vi "Get Default Pressure Units.vi"(8 "error in (no error)":errorcluster, 11 "VISA resource name":refnum<visa-resource-name>) -> (0 "error out":errorcluster, 2 "Default Pressure Units":i32, 3 "VISA resource name out":refnum<visa-resource-name>)   [LabVIEW 2013, in "Fluke 5XXX Series Multicalibrators.lvlib"]
doc: "This VI returns the power-up and reset default pressure display units.\n\nNote:\n\nThis VI is available only for instrument model 5520A with option 700P (pressure modules)."
uses:
  Fluke 5XXX Series Multicalibrators.lvlib
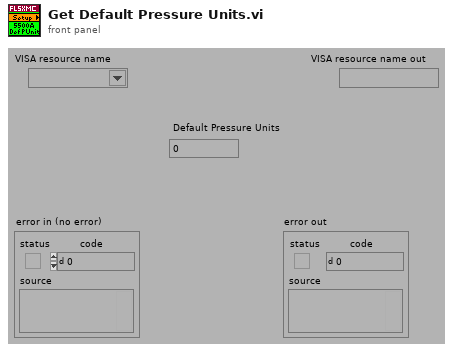
[diagram p1: front panel]
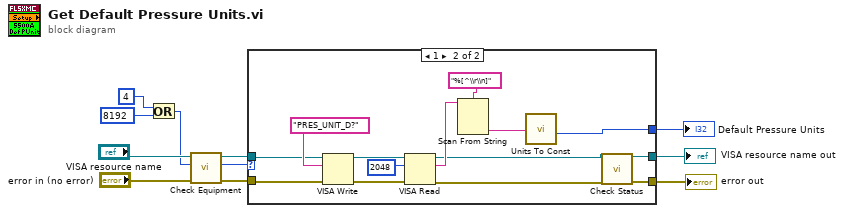
[diagram p0: block diagram]
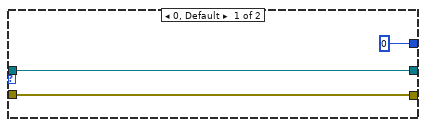
[diagram p2: hidden frame]
diagram:
  n1 = Or(x=4 ("Numeric"), y=8192 ("Numeric")) -> (x .or. y?=w2:i32)
  n2 = call "Check Equipment.vi"("error in (no error)"="error in (no error)", "Bit Mask"=w2, "VISA resource name"="VISA resource name") -> ("error out"=w11:errorcluster, "Present?"=w10:u32, "VISA resource name out"=w9:refnum<visa-resource-name>)  [unwired: 6 in]
  n3 = case shown="1" w10 {
    tunnel: [w14 w22] -> w6
    tunnel: [w13 w21] -> w5
    tunnel: w11 -> [w14 w24]
    tunnel: w9 -> [w13 w23]
    tunnel: [0 w18] -> w1
    frame 0, Default {
    }
    frame 1 {
      n4 = VISA Write(VISA resource name=w23, write buffer="PRES_UNIT_D?", error in (no error)=w24) -> (VISA resource name out=w27:refnum<visa-resource-name>, error out=w26:errorcluster)  [unwired: 1 out]
      n5 = VISA Read(VISA resource name=w27, byte count=u32 2048 ("byte count (0)"), error in (no error)=w26) -> (VISA resource name out=w16:refnum<visa-resource-name>, read buffer=w19:string, error out=w17:errorcluster)  [unwired: 1 out]
      n6 = Scan From String(format string="%[^\\r\\n]", input string=w19) -> (output 1=w15:string)  [unwired: 3 in, 3 out]
      n7 = call "Units To Const.vi"("Units"=w15) -> ("Const"=w18:i32)  [unwired: 10 in]
      n8 = call "Check Status.vi"("VISA resource name"=w16, "error in (no error)"=w17) -> ("VISA resource name out"=w21:refnum<visa-resource-name>, "error out"=w22:errorcluster)  [unwired: 12 in]
    }
  }
  "Default Pressure Units" <- w1
  "VISA resource name out" <- w5
  "error out" <- w6
